vi "Shared Variable Performance Test.vi"() -> ()   [LabVIEW 2021]
panel:
  out "x-y":dbl format="%#_6p"
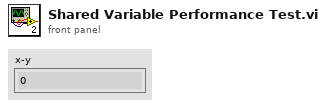
[diagram p1: front panel]
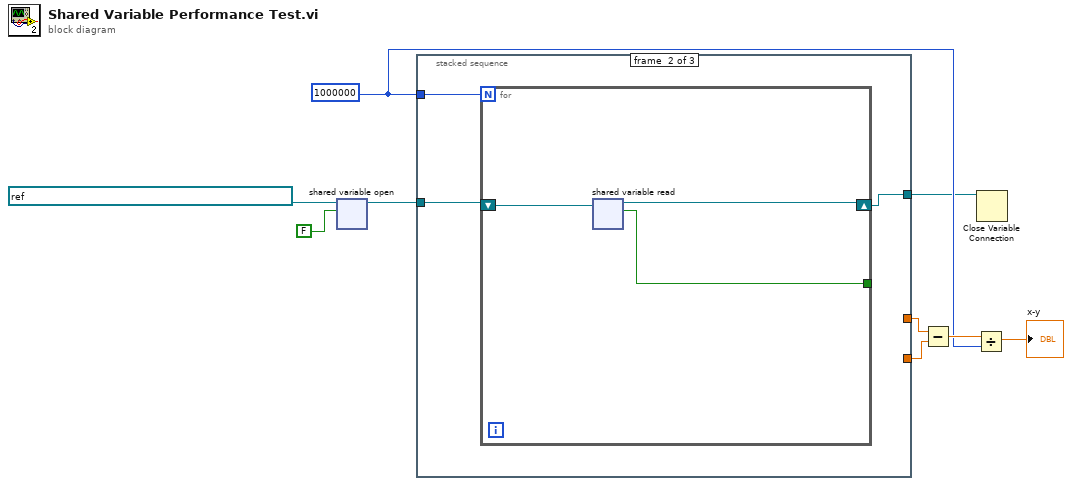
[diagram p0: block diagram]
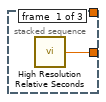
[diagram p2: hidden frame]
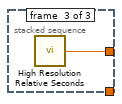
[diagram p3: hidden frame]
diagram:
  w5 = 1000000
  n1 = shared-variable-open(refnum<k21> "ni.var.psp://localhost/Test Shared Variables/Bool" ("shared variable refnum in"), FALSE) -> (w4:refnum<k21>)  [unwired: 2 in, 1 out]
  n2 = stacked-sequence {
    tunnel: [w10 _ _] -> w9
    tunnel: [_ _ w17] -> w8
    tunnel: w5 -> [_ w13 _]
    tunnel: w4 -> [_ w12 _]
    tunnel: [_ w11 _] -> w1
    frame #0 {
      n3 = call <vilib>:"High Resolution Relative Seconds.vi"() -> ("relative seconds"=w10:dbl)
    }
    frame #1 {
      n4 = for {
        N: w13 -> [_]
        shift-right: [w15] -> w11
        shift-left: w12 -> [w16]
        tunnel: [w14] -> _
        n5 = shared-variable-read(w16) -> (w15:refnum<k21>, w14:bool)  [unwired: 1 in, 2 out]
      }
    }
    frame #2 {
      n6 = call <vilib>:"High Resolution Relative Seconds.vi"() -> ("relative seconds"=w17:dbl)
    }
  }
  n7 = Subtract(x=w8, y=w9) -> (x-y=w7:dbl)
  n8 = Divide(x=w7, y=w5) -> (x/y=→"x-y":dbl)
  n9 = Close Variable Connection(11:w1) -> ()  [unwired: 1 in, 1 out]
